vi "Set Drive Mode.vi"(8 "error in (no error)":errorcluster, 10 "Drive Mode":T1, 11 "DC Brick in":refnum<class "DC Brick.lvclass">) -> (0 "error out":errorcluster, 3 "DC Brick out":refnum<class "DC Brick.lvclass">)   [LabVIEW 2011, in "Tinkerforge.lvlib" / "DC Brick.lvclass"]
doc: "This VI sets the drive mode. Possible modes are: * 0 = Drive/Brake * 1 = Drive/Coast\n\nThese modes are different kinds of motor controls.\n\nIn Drive/Brake mode, the motor is always either driving or braking. There is no freewheeling. Advantages are: A more linear correlation between PWM and velocity, more exact accelerations and the possibility to drive with slower velocities.\n\nIn Drive/Coast mode, the motor is always either driving or freewheeling. Advantages are: Less current consumption and less demands on the motor/driver.\n\nThe default value is 0 = Drive/Brake."
uses:
  DC Brick.lvclass
  Type Definitions/Drive Mode.ctl
  Device/Device.lvclass
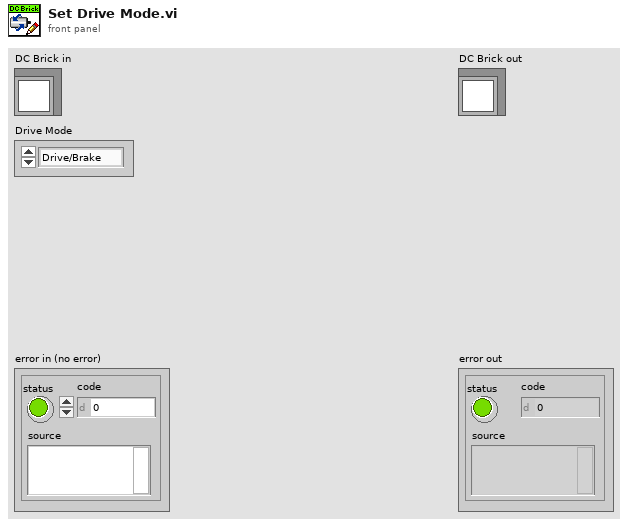
[diagram p1: front panel]
types:
  T1 = typedef "Tinkerforge.lvlib/DC Brick.lvclass/Drive Mode.ctl" = enum16{"Drive/Brake", "Drive/Coast"}
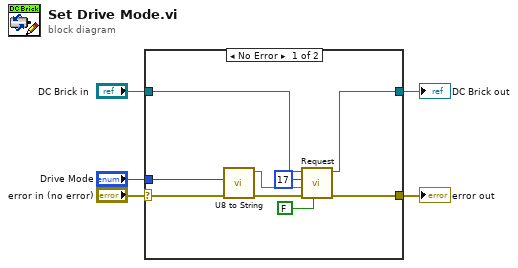
[diagram p0: block diagram]
diagram:
  n1 = case shown="No Error" "error in (no error)" {
    selector: "error in (no error)" -> [w9 w16]
    tunnel: [w10 w16] -> w4
    tunnel: [w13 w15] -> w2
    tunnel: "DC Brick in" -> [w14 w15]
    tunnel: "Drive Mode" -> [w7 _]
    frame No Error {
      n2 = call "U8 to String.vi"("Error In"=w9, "U8"=w7) -> ("Error Out"=w8:errorcluster, "String out"=w6:string)  [unwired: 8 in]
      n3 = call "Request.vi"("Response"=FALSE, "error in (no error)"=w8, "Data"=w6, "Function ID"=u8 17, "Device in"=w14) -> ("error out"=w10:errorcluster, "Device out"=w13:refnum<class "DC Brick.lvclass">)  [unwired: 2 in, 3 out]
    }
    frame Error {
    }
  }
  "error out" <- w4
  "DC Brick out" <- w2
